vi "copy daqmx task.vi"   [LabVIEW 2018]
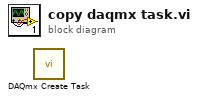
[diagram p0: block diagram]
diagram:
  n1 = call <vilib>:"DAQmx Create Task.vi"() -> ()  [unwired: 14 in, 2 out]
